vi "Owner.vi"(8 "error in (no error)":errorcluster, 11 "Config Element in":refnum<class "Config Element.lvclass">) -> (0 "error out":errorcluster, 2 "Owner":refnum<class "Config Manager.lvclass">, 3 "Config Element out":refnum<class "Config Element.lvclass">)   [LabVIEW 2020, in "CDM-Config.lvlib" / "Config Element.lvclass"]
uses:
  Config Element.lvclass
  Config Element.lvclass/Config Element.ctl
  Config Manager/Config Manager.lvclass
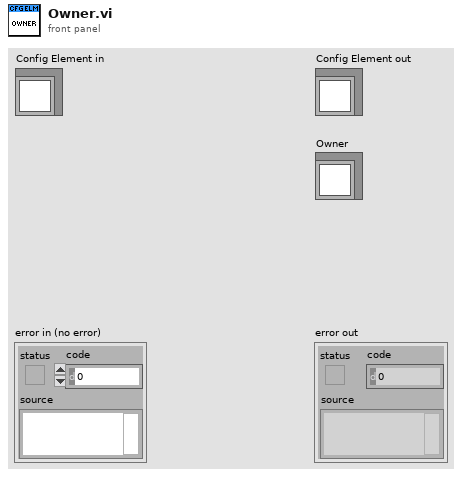
[diagram p1: front panel]
types:
  T1 = typedef "CDM-Config.lvlib/Config Element.lvclass/Ref Data.ctl" = cluster{"Node Info":T2, "Owner":refnum<class>, "Changed":bool, "Name":string, "Value":string, "Meta Data":T3[], "Array":bool}
  T2 = typedef "CDM-Config.lvlib/Node Info.ctl" = cluster{"Index":i32, "Parent":i32, "Children":i32[]}
  T3 = typedef "CDM-Config.lvlib/Meta Data.ctl" = cluster{"Name":string, "Value":string}
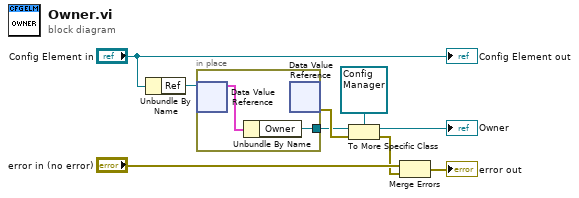
[diagram p0: block diagram]
diagram:
  n1 = Unbundle By Name("Config Element in") -> ("Ref"=w7:refnum<data-value>)
  n2 = in-place {
    in-place-border: [w10] -> w5
    n3 = in-place-dvr #1(w7) -> (w11:T1)  [unwired: 1 out]
    n4 = Unbundle By Name(w11) -> ("Owner"=w10:refnum<class>)
    n5 = in-place-dvr #1() -> (w9:errorcluster)  [unwired: 1 in, 1 out]
  }
  n6 = To More Specific Class(target class=refnum<class "Config Manager.lvclass"> refnum ("CDM-Config.lvlib:Config Manager.lvclass"), reference=w5, error in=w9) -> (specific class reference=→"Owner":refnum<class "Config Manager.lvclass">, error out=w1:errorcluster)
  n7 = Merge Errors("error in (no error)", w1) -> (→"error out":errorcluster)
  "Config Element out" <- "Config Element in"
